vi "longterm_test.vi"() -> ()   [LabVIEW 2017]
uses:
  <vilib>/Math Plots/2D Math Plots/2D Error Bar/2D Error Bar XCtrl/2D Error Bar.xctl
  <vilib>/Math Plots/2D Math Plots/2D Error Bar/2D Error Bar Datatype/2D Error Bar Datatype.lvclass
  <vilib>/Math Plots/2D Math Plots/2D Error Bar/2D Error Bar Datatype/Public/Plot Helper (Fixed).vi
panel:
  out "temperature":T1(graph)=[{"seconds since 1Jan1904"=timestamp(3811629259.5421824 s since 1904-01-01), "mean[ps]"=81.52453053079984}, {"seconds since 1Jan1904"=timestamp(3811629559.5649886 s since 1904-01-01), "mean[ps]"=83.40520185718381}]
  in  "stop":bool
  out "误差线":refnum<class "2D Plot Datatype.lvclass">[](xcontrol)
  out "sigma[ps]":dbl=22.57071615137417 format="%0.2f"
  out "Sigma":T1(graph)=[{"seconds since 1Jan1904"=timestamp(3811629259.5421824 s since 1904-01-01), "mean[ps]"=24.445797392886654}, {"seconds since 1Jan1904"=timestamp(3811629559.5649886 s since 1904-01-01), "mean[ps]"=22.57071615137417}]
  in  "times":i32=4
  out "mean[ps]":dbl=83.40520185718381 format="%0.2f"
  out "seconds since 1Jan1904":timestamp=timestamp(3811629559.5649886 s since 1904-01-01)
  out "Counter":i32=2
  out "Mean":T1(graph)=[{"seconds since 1Jan1904"=timestamp(3811629259.5421824 s since 1904-01-01), "mean[ps]"=81.52453053079984}, {"seconds since 1Jan1904"=timestamp(3811629559.5649886 s since 1904-01-01), "mean[ps]"=83.40520185718381}]
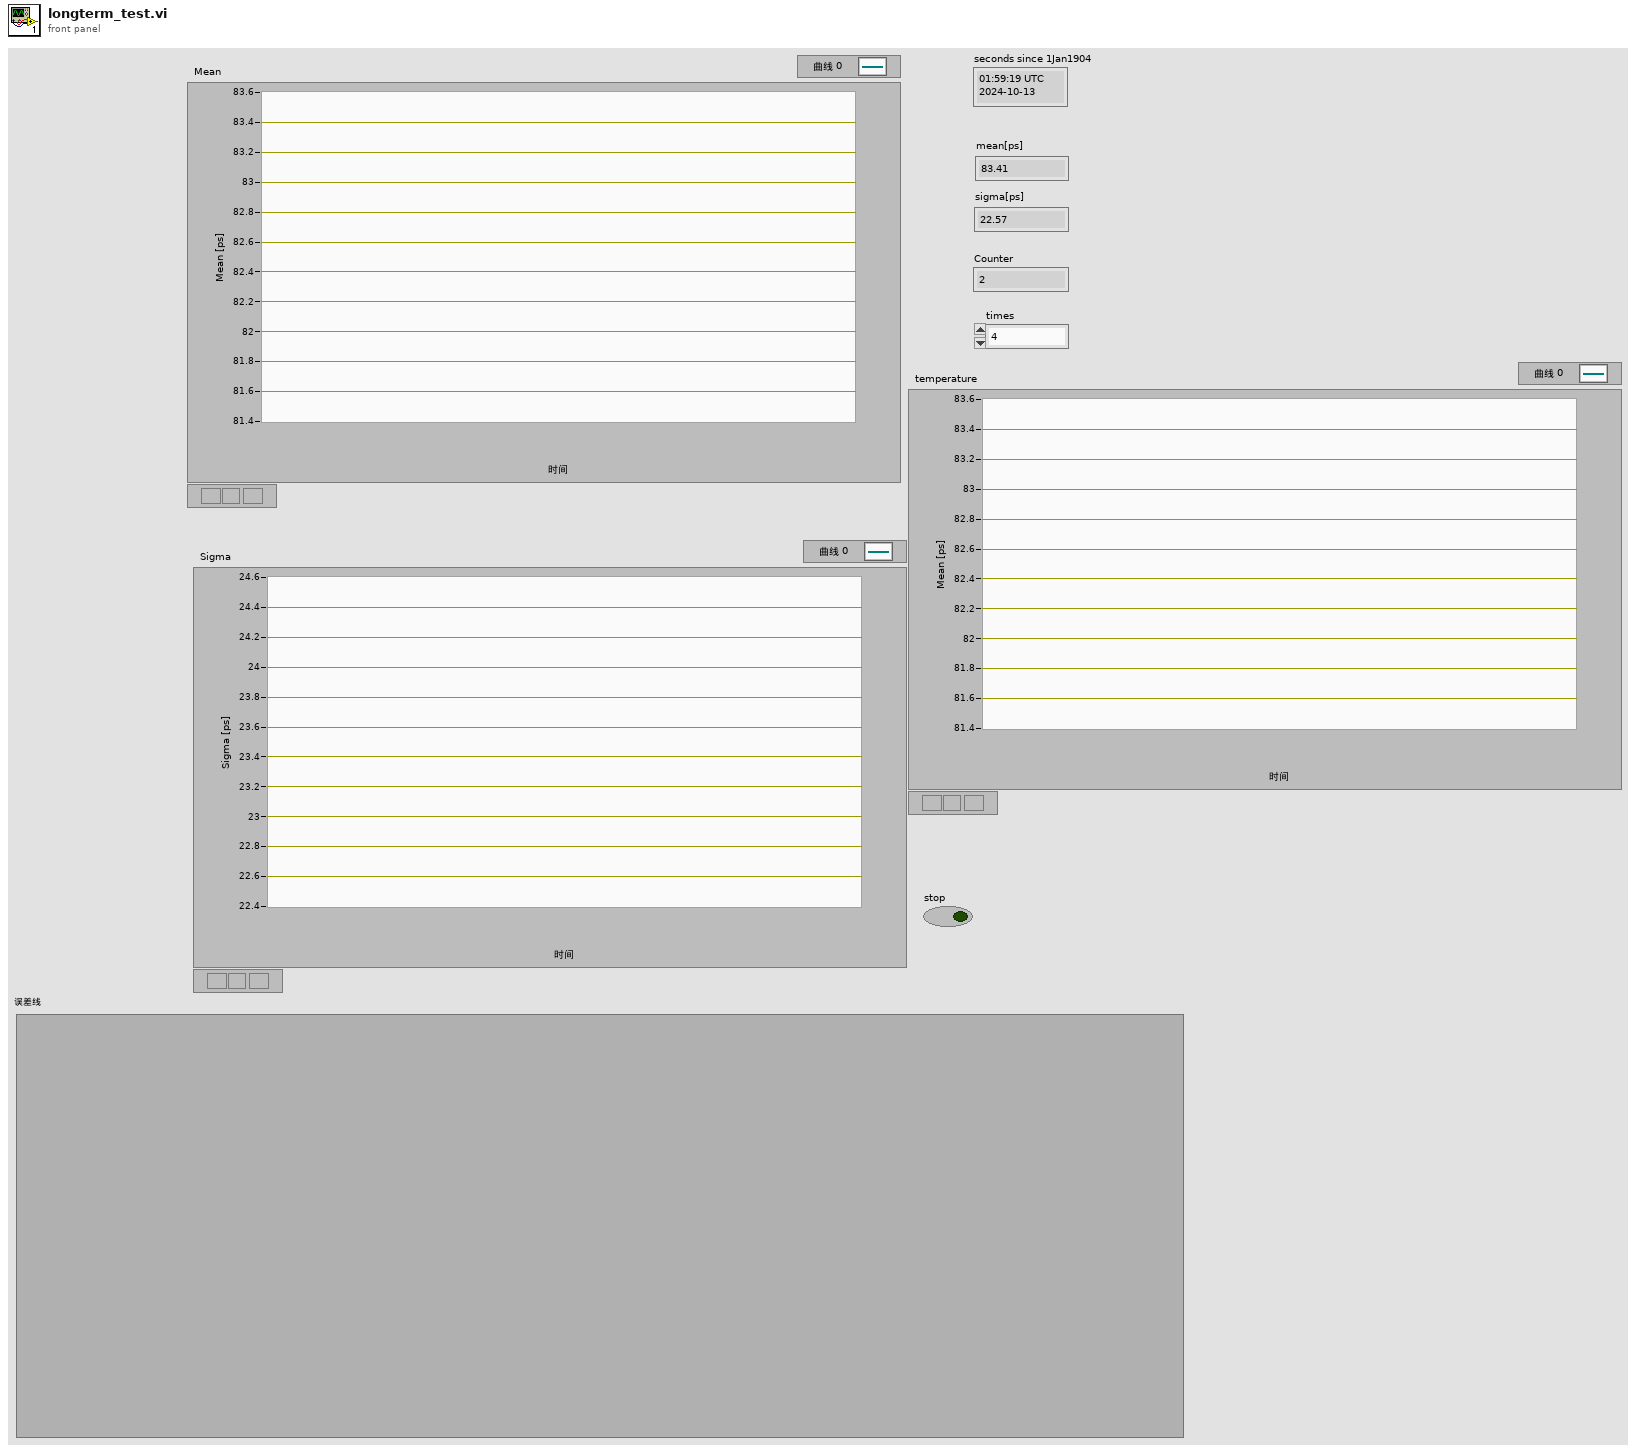
[diagram p1: front panel]
types:
  T1 = cluster{"seconds since 1Jan1904":timestamp, "mean[ps]":dbl}[]
  T2 = cluster{"seconds since 1Jan1904":timestamp, "mean[ps]":dbl}
  T3 = cluster{"seconds since 1Jan1904":timestamp, "standard deviation[ps]":dbl}
  T4 = cluster{"seconds since 1Jan1904":timestamp, "Tc[℃]":dbl}
  T5 = cluster{"seconds since 1Jan1904":timestamp, "Vcc_int[mV]":dbl}
  T6 = cluster{"seconds since 1Jan1904":timestamp, "standard deviation[ps]":dbl}[]
  T7 = cluster{"seconds since 1Jan1904":timestamp, "Tc[℃]":dbl}[]
  T8 = cluster{"seconds since 1Jan1904":timestamp, "Vcc_int[mV]":dbl}[]
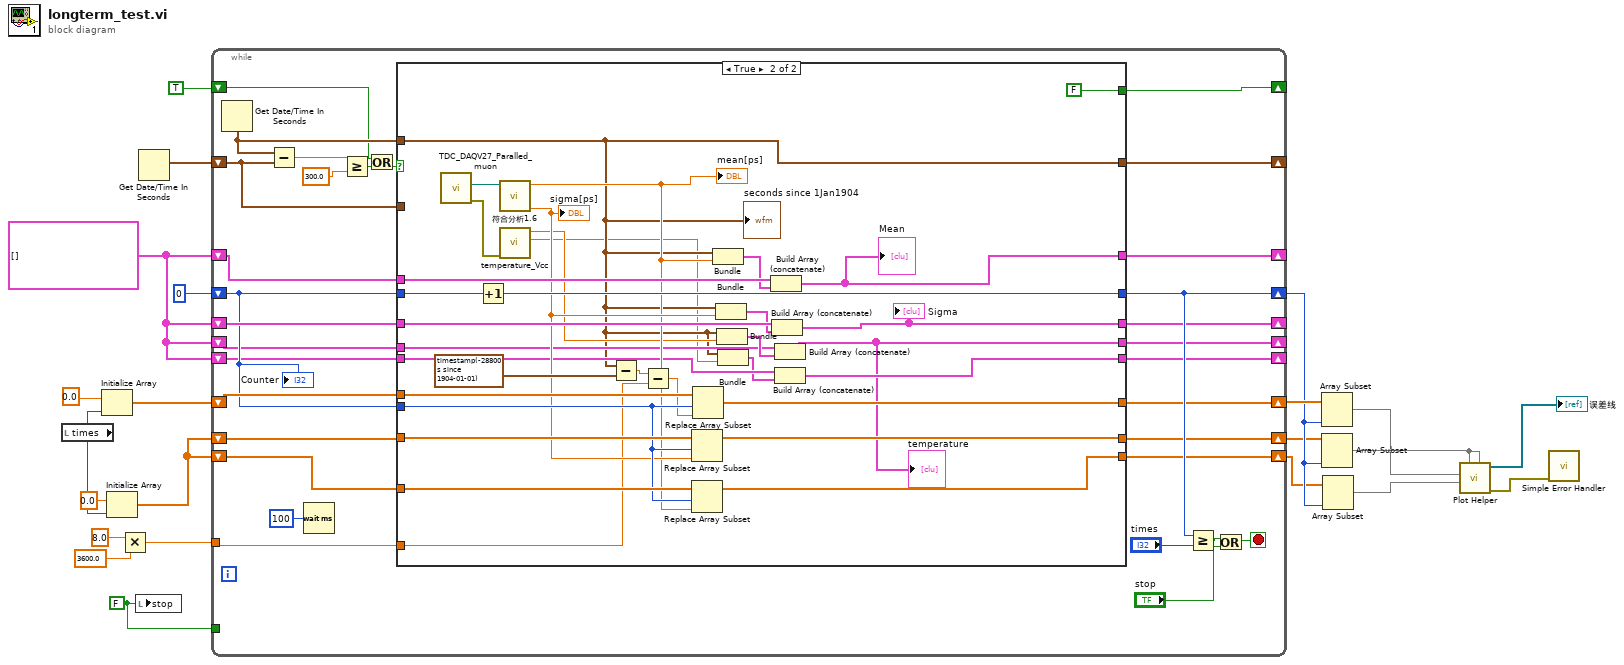
[diagram p0: block diagram]
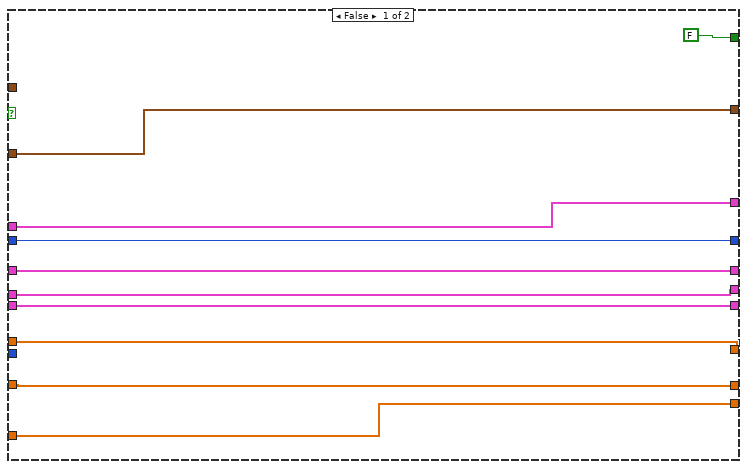
[diagram p2: hidden frame]
diagram:
  w2 = FALSE ("stop")
  w1 = T1 []
  n1 = local read "times"() -> (w18:i32)
  n2 = Initialize Array(0.0 ("mean[ps]"), w18) -> (w19:dbl[])
  n3 = Initialize Array(0.0 ("mean[ps]"), w18) -> (w17:dbl[])
  n4 = Multiply(x=8.0, y=3600.0) -> (x*y=w12:dbl)
  n5 = local write "stop"(w2) -> ()
  n6 = Get Date/Time In Seconds() -> (seconds since 1Jan1904=w22:timestamp)
  n7 = while {
    shift-right: [w49] -> _
    shift-left: w22 -> [w50]
    shift-right: [w47] -> w6
    shift-left: 0 -> [w36]
    shift-right: [w42] -> _
    shift-left: TRUE -> [w43]
    shift-right: [w40] -> _
    shift-left: w1 -> [w41]
    shift-right: [w38] -> _
    shift-left: w1 -> [w39]
    shift-right: [w33] -> w7
    shift-left: w19 -> [w37]
    shift-right: [w32] -> w4
    shift-left: w17 -> [w35]
    shift-right: [w30] -> w5
    shift-left: w17 -> [w34]
    tunnel: w12 -> [w31]
    tunnel: w2 -> [_]
    shift-right: [w25] -> _
    shift-left: w1 -> [w26]
    shift-right: [w23] -> _
    shift-left: w1 -> [w24]
    stop <- w28 stop-if-true
    n8 = Get Date/Time In Seconds() -> (seconds since 1Jan1904=w48:timestamp)
    n9 = Subtract(x=w48, y=w50) -> (x-y=w53:dbl)
    n10 = Wait (ms)(milliseconds to wait=u32 100 ("等待时间（毫秒）")) -> ()  [unwired: 1 out]
    n11 = Greater Or Equal?(x=w53, y=300.0) -> (x >= y?=w51:bool)
    n12 = Or(x=w43, y=w51) -> (x .or. y?=w44:bool)
    n13 = case shown="True" w44 {
      tunnel: w50 -> [w63 _]
      tunnel: [w63 w70] -> w49
      tunnel: w48 -> [_ w70]
      tunnel: w36 -> [w62 w96]
      tunnel: [w62 w84] -> w47
      tunnel: [FALSE FALSE] -> w42
      tunnel: w41 -> [w60 w94]
      tunnel: [w60 w93] -> w40
      tunnel: w39 -> [w59 w91]
      tunnel: [w59 w89] -> w38
      tunnel: w37 -> [w58 w88]
      tunnel: w36 -> [_ w83]
      tunnel: w35 -> [w57 w86]
      tunnel: w34 -> [w56 w85]
      tunnel: [w58 w80] -> w33
      tunnel: [w57 w76] -> w32
      tunnel: [w56 w75] -> w30
      tunnel: w31 -> [_ w79]
      tunnel: w26 -> [w55 w72]
      tunnel: [w55 w64] -> w25
      tunnel: w24 -> [w54 w71]
      tunnel: [w54 w67] -> w23
      frame False {
      }
      frame True {
        n14 = call "TDC_DAQV27_Paralled_muon.vi"() -> ("error out 3"=w65:errorcluster, "appended path"=w66:path)  [unwired: 9 in, 1 out]
        n15 = Increment(x=w96) -> (x+1=w84:i32)
        n16 = call "符合分析1.6.vi"("file path (dialog if empty)"=w66) -> ("standard deviation[ps]"=w82:dbl, "mean[ps]"=w81:dbl)  [unwired: 6 in, 3 out]
        "mean[ps]" <- w81
        "sigma[ps]" <- w82
        n17 = call "temperature_Vcc.vi"("error in (no error)"=w65) -> ("Vcc_int[mV]"=w69:dbl, "Tc[℃]"=w73:dbl)  [unwired: 8 in, 1 out]
        n18 = Subtract(x=w70, y=timestamp(-28800 s since 1904-01-01) ("seconds since 1Jan1904")) -> (x-y=w78:dbl)
        n19 = Subtract(x=w78, y=w79) -> (x-y=w77:dbl)
        n20 = Replace Array Subset(array=w86, new element=w82, index=w83) -> (w76:dbl[])
        n21 = Replace Array Subset(array=w85, new element=w81, index=w83) -> (w75:dbl[])
        n22 = Replace Array Subset(array=w88, new element=w77, index=w83) -> (w80:dbl[])
        n23 = Bundle("seconds since 1Jan1904"=w70, "mean[ps]"=w81) -> (w92:T2)  [unwired: 1 in]
        n24 = Bundle("seconds since 1Jan1904"=w70, "standard deviation[ps]"=w82) -> (w90:T3)  [unwired: 1 in]
        n25 = Bundle("seconds since 1Jan1904"=w70, "Tc[℃]"=w73) -> (w74:T4)  [unwired: 1 in]
        n26 = Bundle("seconds since 1Jan1904"=w70, "Vcc_int[mV]"=w69) -> (w68:T5)  [unwired: 1 in]
        n27 = Build Array (concatenate)(w94, w92) -> (w93:T1)
        "Mean" <- w93
        n28 = Build Array (concatenate)(w91, w90) -> (w89:T6)
        "Sigma" <- w89
        n29 = Build Array (concatenate)(w72, w74) -> (w64:T7)
        "temperature" <- w64
        n30 = Build Array (concatenate)(w71, w68) -> (w67:T8)
        "seconds since 1Jan1904" <- w70
      }
    }
    n31 = Greater Or Equal?(x=w47, y="times") -> (x >= y?=w29:bool)
    n32 = Or(x=w29, y="stop") -> (x .or. y?=w28:bool)
    "Counter" <- w36
  }
  n33 = Array Subset(array=w7, length=w6) -> (w10:dbl[])  [unwired: 1 in]
  n34 = Array Subset(array=w4, length=w6) -> (w11:dbl[])  [unwired: 1 in]
  n35 = Array Subset(array=w5, length=w6) -> (w3:dbl[])  [unwired: 1 in]
  n36 = call-poly <vilib>:"Plot Helper.vi"("error b vector"=w11, "error a vector"=w11, "y vector"=w3, "x vector"=w10) -> ("error out"=w8:errorcluster, "2D Plot Class Obj Array out"=→"误差线":refnum<class "2D Plot Datatype.lvclass">[])  [unwired: 2 in, 4 out]
  n37 = call <vilib>:"Simple Error Handler.vi"("error in (no error)"=w8) -> ()  [unwired: 4 in, 5 out]
